vi "automatic_wait.vi"(5 "change_in_event":refnum<user-event>, 7 "waitgroup":T1, 8 "error in (no error)":errorcluster, 11 "data":variant) -> (0 "error out":errorcluster)   [LabVIEW 2015, in "example_01.lvlib"]
uses:
  example_01.lvlib
  <userlib>/antonio-alexander/lv-waitgroup/public/_controls/api_waitgroup.ctl
  lv-recipe-machine/public/_controls/change.ctl
  _controls/step_data.ctl
  _controls/automatic_steps.ctl
  lv-recipe-machine/lv-recipe-machine.lvlib
  <userlib>/antonio-alexander/lv-waitgroup/lv-waitgroup.lvlib
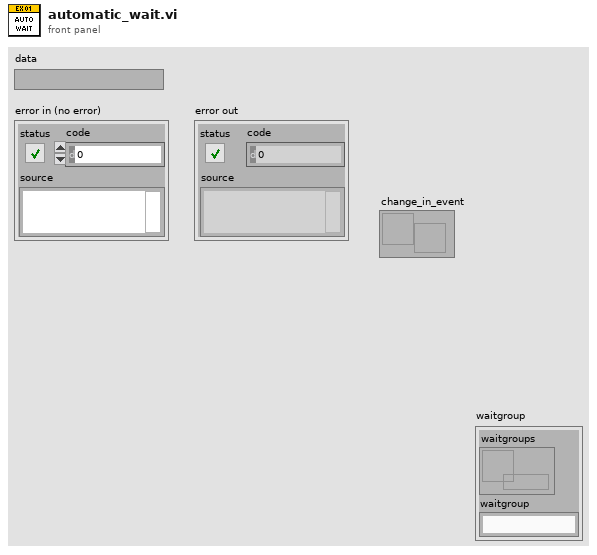
[diagram p1: front panel]
types:
  T1 = typedef "lv-waitgroup.lvlib/api_waitgroup.ctl" = cluster{"waitgroups":refnum<data-value>, "waitgroup":string}
  T2 = typedef "example_01.lvlib/automatic_steps.ctl" = enum16{"<automatic_step>", "auto_initialize", "auto_test_random", "auto_test_comparison", "auto_wait", "auto_complete_continue", "auto_complete_fail", "auto_complete_finish", "<null>"}
  T3 = typedef "example_01.lvlib/step_data.ctl" = cluster{"data":variant, "step":string}
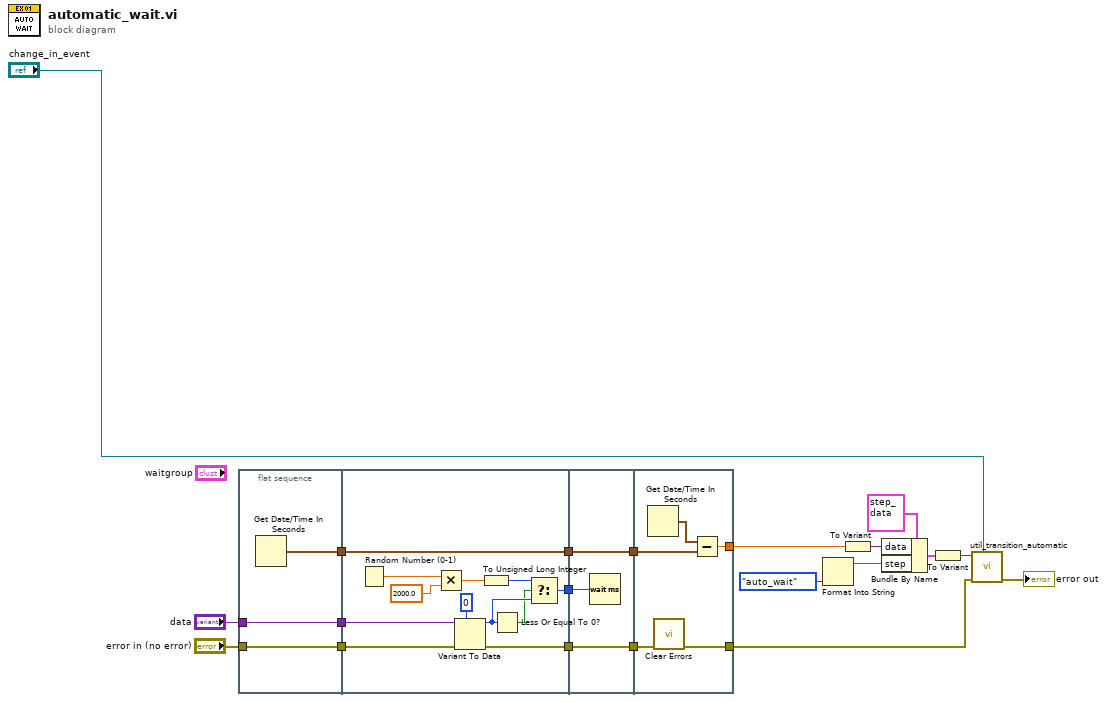
[diagram p0: block diagram]
diagram:
  n1 = flat-sequence {
    tunnel: "data" -> [w23]
    tunnel: "error in (no error)" -> [w22]
    tunnel: [w23] -> w20
    tunnel: [w22] -> w19
    tunnel: [w21] -> w18
    tunnel: w20 -> [w28]
    tunnel: w19 -> [w29]
    tunnel: w18 -> [w35]
    tunnel: [w35] -> w17
    tunnel: [w27] -> w16
    tunnel: [w24] -> w15
    tunnel: w17 -> [w38]
    tunnel: [w38] -> w14
    tunnel: w16 -> [w37]
    tunnel: [w36] -> w13
    tunnel: w15 -> [w36]
    tunnel: w14 -> [w42]
    tunnel: [w41] -> w9
    tunnel: [w40] -> w2
    tunnel: w13 -> [w39]
    frame #0 {
      n2 = Get Date/Time In Seconds() -> (seconds since 1Jan1904=w21:timestamp)
    }
    frame #1 {
      n3 = Random Number (0-1)() -> (number: 0 to 1=w31:dbl)
      n4 = Multiply(x=w31, y=2000.0) -> (x*y=w33:dbl)
      n5 = Variant To Data(error in=w29, type=u32 0, Variant=w28) -> (data=w26:u32, error out=w24:errorcluster)
      n6 = To Unsigned Long Integer(number=w33) -> (unsigned 32bit integer=w34:u32)
      n7 = Less Or Equal To 0?(x=w26) -> (x <= 0?=w25:bool)
      n8 = Select(t=w34, s=w25, f=w26) -> (s? t:f=w27:u32)
    }
    frame #2 {
      n9 = Wait (ms)(milliseconds to wait=w37) -> ()  [unwired: 1 out]
    }
    frame #3 {
      n10 = Get Date/Time In Seconds() -> (seconds since 1Jan1904=w43:timestamp)
      n11 = call <vilib>:"Clear Errors.vi"("error in (no error)"=w39) -> ("error out"=w40:errorcluster)  [unwired: 5 in, 1 out]
      n12 = Subtract(x=w43, y=w42) -> (x-y=w41:dbl)
    }
  }
  n13 = Format Into String(automatic_steps."auto_wait" ("automatic_steps")) -> (resulting string=w11:string)  [unwired: 3 in, 1 out]
  n14 = To Variant(anything=w9) -> (Variant=w10:variant)
  n15 = Bundle By Name(cluster=T3 {"data"=variant, "step"=""}, "data"=w10, "step"=w11) -> (w7:T3)
  n16 = To Variant(anything=w7) -> (Variant=w4:variant)
  n17 = call "util_transition_automatic.vi"("change_in_event"="change_in_event", "error in (no error)"=w2, "data"=w4) -> ("error out"=→"error out":errorcluster)  [unwired: 8 in]
